vi "ukol2.vi"() -> ()   [LabVIEW 2022 SP3]
panel:
  out "Numeric":dbl
  out "32bit integer":i32[][](array[numeric])
  out "Array 3":dbl[](array[numeric])
  in  "Array 2":dbl[](array[numeric])
  in  "Array":dbl[](array[numeric])
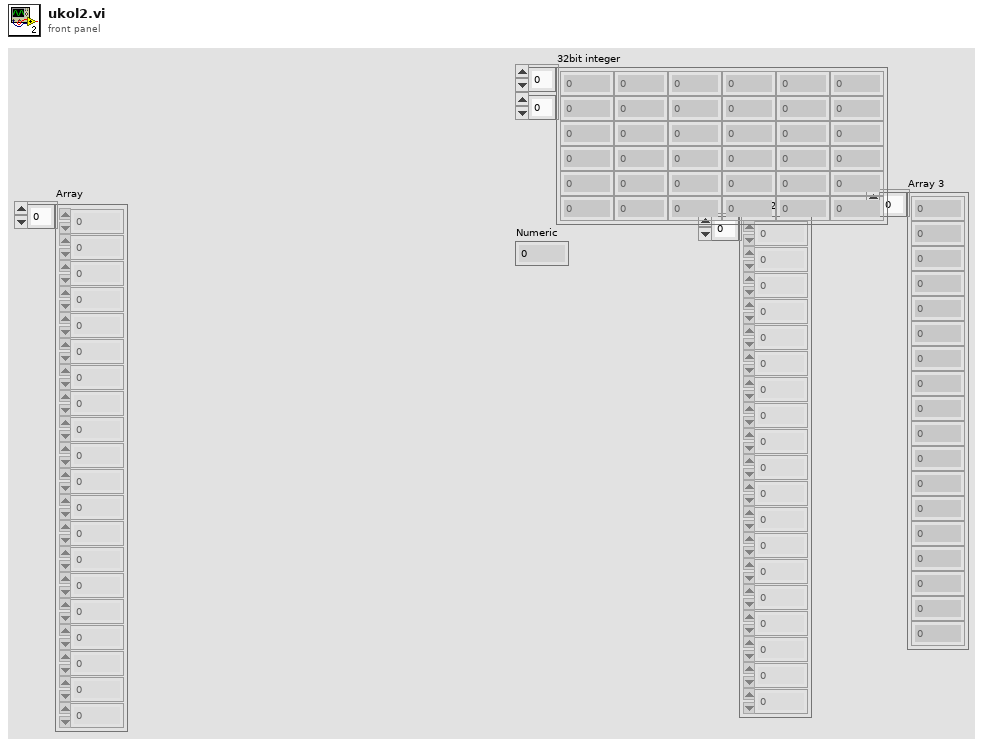
[diagram p1: front panel]
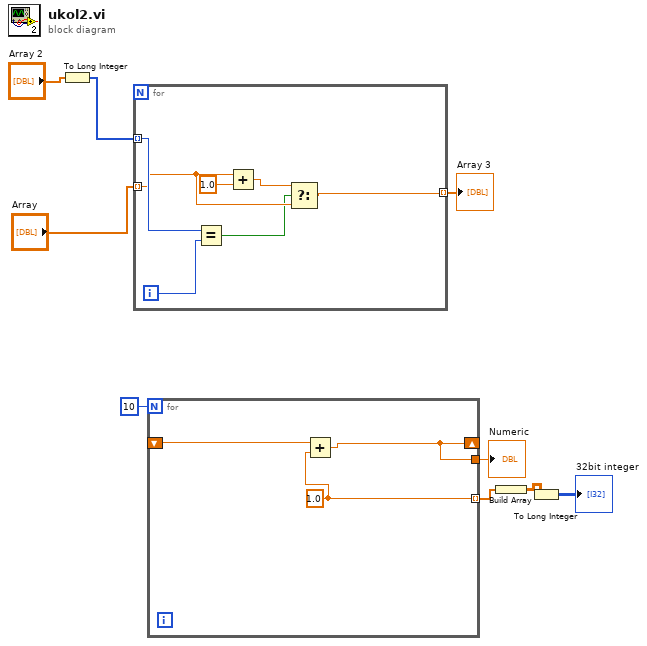
[diagram p0: block diagram]
diagram:
  n1 = To Long Integer(number="Array 2") -> (32bit integer=w8:i32[])
  n2 = for {
    tunnel: w8 -> [w15] mode=indexing
    tunnel: "Array" -> [w12] mode=indexing
    tunnel: [w10] -> w6 mode=indexing
    i -> [w16]
    n3 = Equal?(x=w15, y=w16) -> (x = y?=w11:bool)
    n4 = Add(x=w12, y=1.0) -> (x+y=w13:dbl)
    n5 = Select(t=w13, s=w11, f=w12) -> (s? t:f=w10:dbl)
  }
  "Array 3" <- w6
  n6 = for {
    N: 10 -> [_]
    tunnel: [w19] -> w2 mode=indexing
    shift-right: [w17] -> _
    shift-left: _ -> [w18]
    tunnel: [w17] -> w1
    w19 = 1.0 ("element")
    n7 = Add(x=w18, y=w19) -> (x+y=w17:dbl)
  }
  "Numeric" <- w1
  n8 = Build Array(w2) -> (w3:dbl[][])
  n9 = To Long Integer(number=w3) -> (32bit integer=→"32bit integer":i32[][])
